vi "recv_packet.vi"(8 "error in (no error)":errorcluster, 11 "TCP Network Connection in":refnum<k5>) -> (0 "error out":errorcluster, 2 "w5500_pck":T1, 3 "TCP Network Connection out":refnum<k5>)   [LabVIEW 2021]
uses:
  typedefs/w5500_pck.ctl
  typedefs/w5500_cmd.ctl
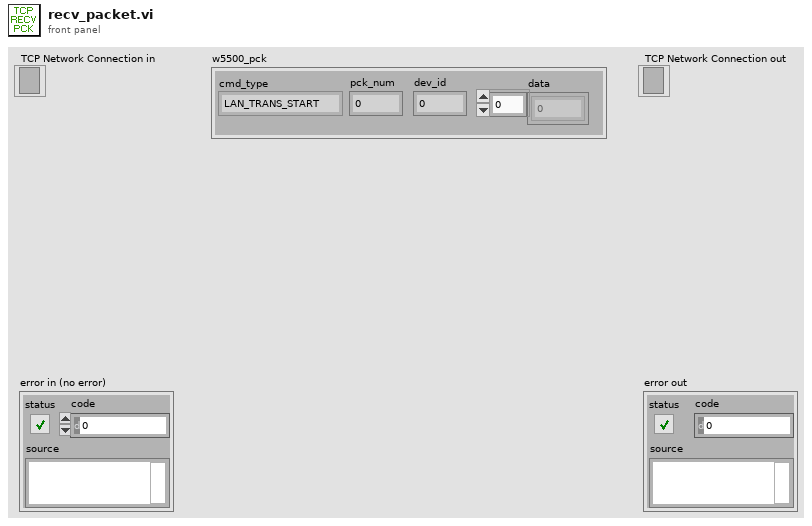
[diagram p1: front panel]
types:
  T1 = typedef "w5500_pck.ctl" = cluster{"cmd_type":T2, "pck_num":u32, "dev_id":u32, "data":u8[]}
  T2 = typedef "w5500_cmd.ctl" = enum32{"LAN_TRANS_START", "LAN_DATA_SZ", "LAN_CHUNK_SEND", "LAN_CHUNK_ACK", "LAN_DEVS_INFO", "LAN_DEVS_NUM", "LAN_DEVS_EXS", "LAN_DEVS_ACK", "LAN_CMD_ACK", "LAN_CMD_FIN", "LAN_SND_STAT", "LAN_REQ_STAT", "LAN_ANS_STAT", "LAN_ERR_STAT", "LAN_SETT_SET", "LAN_SETT_GET", "LAN_SETT_ACK", "LAN_SETT_ERR"}
  T3 = enum16{"big-endian, network order", "native, host order", "little-endian"}
  T4 = enum16{"Standard", "Buffered", "CRLF", "Immediate"}
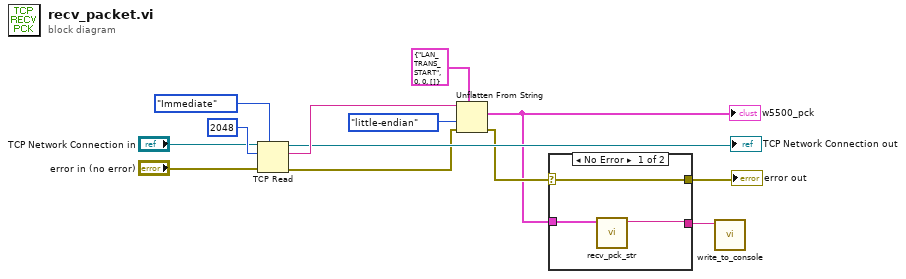
[diagram p0: block diagram]
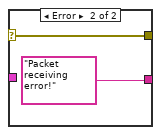
[diagram p2: hidden frame]
diagram:
  n1 = TCP Read(connection ID="TCP Network Connection in", bytes to read=2048, error in (no error)="error in (no error)", 7:T4."Immediate" ("mode (standard)")) -> (connection ID out=→"TCP Network Connection out":refnum<k5>, data out=w11:string, error out=w5:errorcluster)  [unwired: 1 in]
  n2 = Unflatten From String(type=T1 {"cmd_type"=enum."LAN_TRANS_START", "pck_num"=0, "dev_id"=0, "data"=[]} ("w5500_pck"), binary string=w11, byte order (0:big-endian, network order)=T3."little-endian", error in (no error)=w5) -> (value=w1:T1, error out=w3:errorcluster)  [unwired: 1 in, 1 out]
  "w5500_pck" <- w1
  n3 = case shown="No Error" w3 {
    selector: w3 -> [w16 w17]
    tunnel: [w16 w17] -> w2
    tunnel: [w15 "Packet receiving error!"] -> w4
    tunnel: w1 -> [w14 _]
    frame No Error {
      n4 = call "recv_pck_str.vi"("inp_pck"=w14) -> ("res_str"=w15:string)  [unwired: 10 in]
    }
    frame Error {
    }
  }
  "error out" <- w2
  n5 = call "write_to_console.vi"("input_str"=w4) -> ()  [unwired: 10 in, 1 out]
